vi "_Veritech_LVCM_Provider_Shutdown.vi"(8 "error in (no error)":errorcluster, 10 "Is LV Exiting?":bool, 11 "Project Refnum":refnum<vi>) -> (0 "error out":errorcluster)   [LabVIEW 2014]
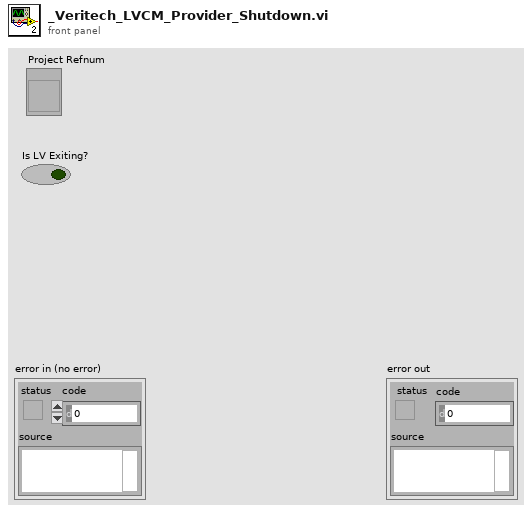
[diagram p1: front panel]
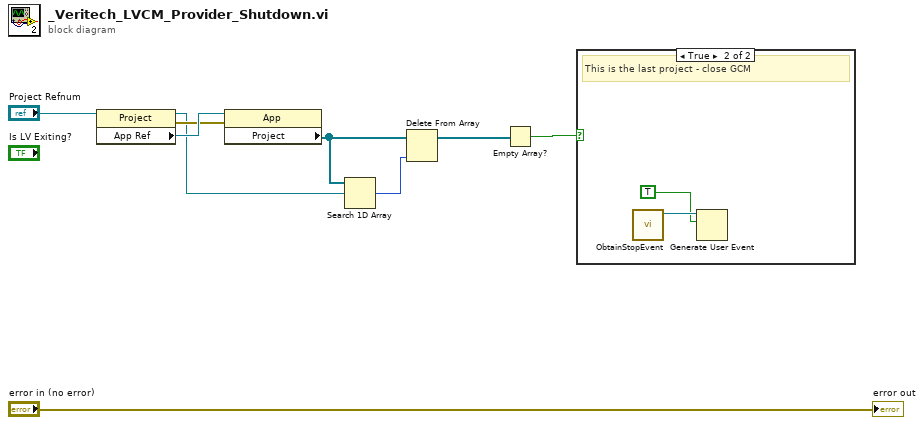
[diagram p0: block diagram]
diagram:
  n1 = property class="Project"(reference="Project Refnum") -> (reference out=w4:refnum<vi>, error out=w6:errorcluster, "App Ref"=w7:refnum<vi>)  [unwired: 1 in]
  n2 = property class="App"(reference=w7, error in=w6) -> ("Project"=w2:refnum<vi>[])  [unwired: 2 out]
  n3 = Search 1D Array(1D array=w2, element=w4) -> (index of element=w3:i32)  [unwired: 1 in]
  n4 = Delete From Array(array=w2, index=w3) -> (array with subset deleted=w1:refnum<vi>[])  [unwired: 1 in, 1 out]
  n5 = Empty Array?(array=w1) -> (empty?=w5:bool)
  n6 = case shown="True" w5 {
    frame False {
      # "There are still opened projects"
    }
    frame True {
      # "This is the last project - close GCM"
      n7 = call "ObtainStopEvent.vi"() -> ("StopEvent"=w11:refnum<user-event>)  [unwired: 11 in]
      n8 = Generate User Event(user event=w11, event data cluster=TRUE ("event data")) -> ()  [unwired: 2 in, 2 out]
    }
  }
  "error out" <- "error in (no error)"
